vi "SeperateNegativePositiveTime.vi"(11 "TimePlotData":T1[](array[typedef])) -> (0 "Negative TimePlotData":T1[](array[typedef]), 3 "Positive TimePlotData":T1[](array[typedef]))   [LabVIEW 2014]
doc: "Separates timing plot data into two arrays depending on whether the values are greater or less than relative zero."
uses:
  Controls/TimingPlotData.ctl
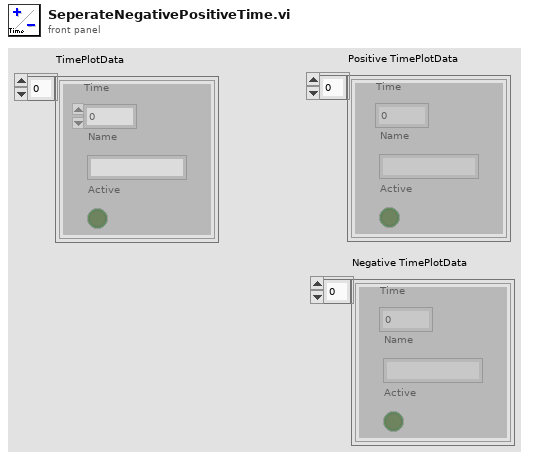
[diagram p1: front panel]
types:
  T1 = typedef "TimingPlotData.ctl" = cluster{"Time":dbl, "Name":string, "Active":bool}
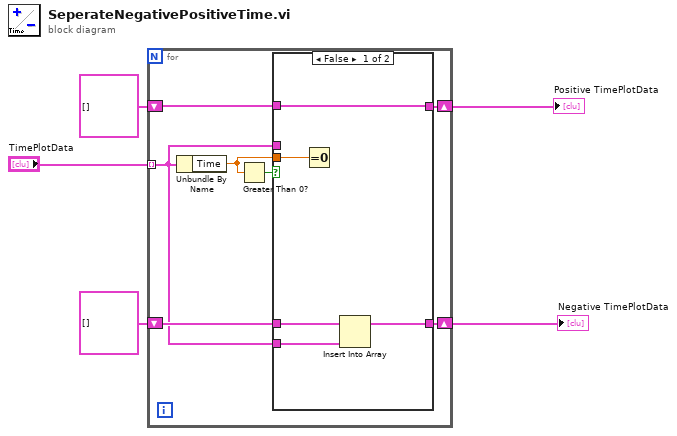
[diagram p0: block diagram]
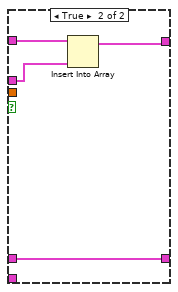
[diagram p2: hidden frame]
diagram:
  n1 = for {
    tunnel: "TimePlotData" -> [w6] mode=indexing
    shift-right: [w10] -> w4
    shift-left: T1[] [] -> [w11]
    shift-right: [w8] -> w3
    shift-left: T1[] [] -> [w9]
    n2 = Unbundle By Name(w6) -> ("Time"=w7:dbl)
    n3 = Greater Than 0?(x=w7) -> (x > 0?=w12:bool)
    n4 = case shown="False" w12 {
      tunnel: w11 -> [w15 w21]
      tunnel: [w14 w21] -> w10
      tunnel: [w17 w19] -> w8
      tunnel: w9 -> [w17 w20]
      tunnel: w6 -> [_ w18]
      tunnel: w7 -> [w16 _]
      tunnel: w6 -> [w13 _]
      frame False {
        n5 = Equal To 0?(x=w16) -> ()  [unwired: 1 out]
        n6 = Insert Into Array(array=w15, new element=w13) -> (w14:T1[])  [unwired: 1 in]
      }
      frame True {
        n7 = Insert Into Array(array=w20, new element=w18) -> (w19:T1[])  [unwired: 1 in]
      }
    }
  }
  "Positive TimePlotData" <- w3
  "Negative TimePlotData" <- w4
